vi "_Node.vi"(1 "TagDB Node (in)":T1) -> (0 "TagDB Node":T1)   [LabVIEW 2014, in "TagDB(dev).lvlib"]
uses:
  TagDB(dev).lvlib
  tagDB_Def.ctl
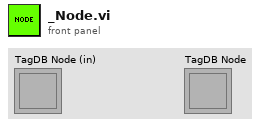
[diagram p1: front panel]
types:
  T1 = typedef "TagDB(dev).lvlib/tagDB_Def.ctl" = refnum<k1>
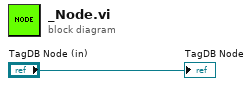
[diagram p0: block diagram]
diagram:
  "TagDB Node" <- "TagDB Node (in)"
